vi "Read Application.vi"(8 "error in (no error)":errorcluster, 11 "TestRunner in":refnum<class "TestRunner.lvclass">) -> (0 "error out":errorcluster, 2 "Application":refnum<vi>, 3 "TestRunner out":refnum<class "TestRunner.lvclass">)   [LabVIEW 2019, in "UnitTestEngine.lvlib" / "TestRunner.lvclass"]
uses:
  TestRunner.lvclass
  TestRunner.lvclass/TestRunner.ctl
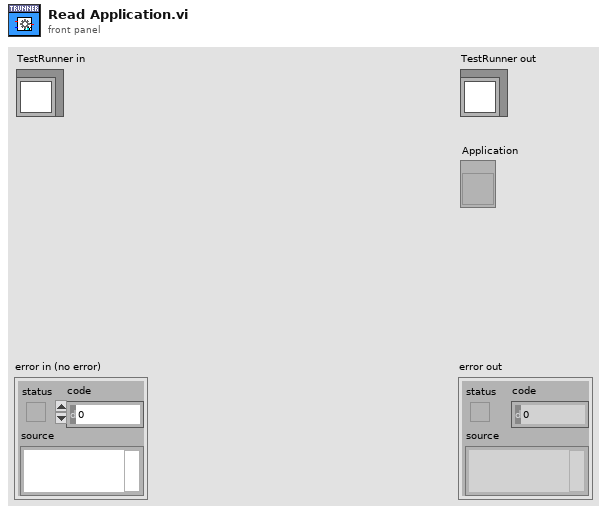
[diagram p1: front panel]
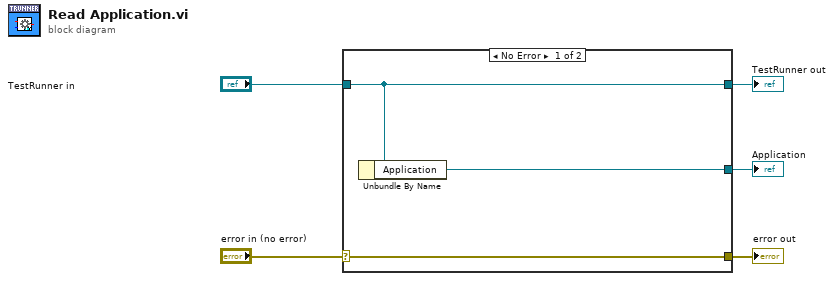
[diagram p0: block diagram]
diagram:
  n1 = case shown="No Error" "error in (no error)" {
    selector: "error in (no error)" -> [w8 w9]
    tunnel: [w8 w9] -> w4
    tunnel: [w7 w10] -> w2
    tunnel: "TestRunner in" -> [w7 w10]
    tunnel: [w6 _] -> w1
    frame No Error {
      n2 = Unbundle By Name(w7) -> ("Application"=w6:refnum<vi>)
    }
    frame Error {
    }
  }
  "error out" <- w4
  "TestRunner out" <- w2
  "Application" <- w1
